vi "_exclude Event Structure Ref.vi"(1 "Part References":T2) -> (0 "NaN/Path/Refnum?":T1)   [LabVIEW 2014]
uses:
  <resource>/dialog/QuickDrop/plugins/_JKI State Machine Helper.llb/Part References -- Cluster__JKI_State_Machine_Helper.ctl
  <resource>/dialog/QuickDrop/plugins/_JKI State Machine Helper.llb/JKI SM__JKI_State_Machine_Helper.lvclass
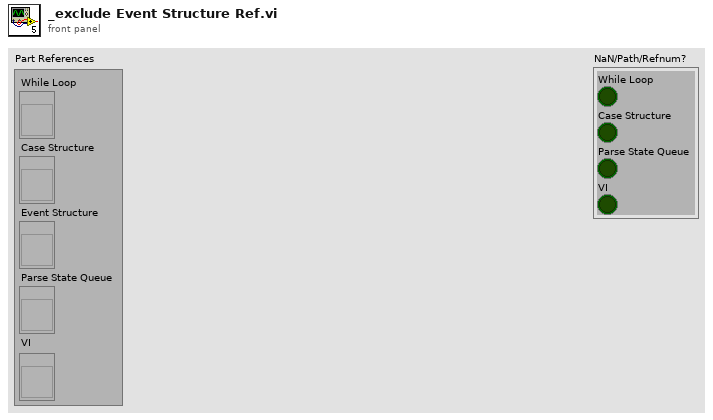
[diagram p1: front panel]
types:
  T1 = cluster{"While Loop":bool, "Case Structure":bool, "Parse State Queue":bool, "VI":bool}
  T2 = typedef "JKI State Machine API__JKI_State_Machine_Helper.lvlib/JKI SM__JKI_State_Machine_Helper.lvclass/Part References -- Cluster__JKI_State_Machine_Helper.ctl" = cluster{"While Loop":refnum<vi>, "Case Structure":refnum<vi>, "Event Structure":refnum<vi>, "Parse State Queue":refnum<vi>, "VI":refnum<vi>}
  T3 = cluster{"While Loop":refnum<vi>, "Case Structure":refnum<vi>, "Parse State Queue":refnum<vi>, "VI":refnum<vi>}
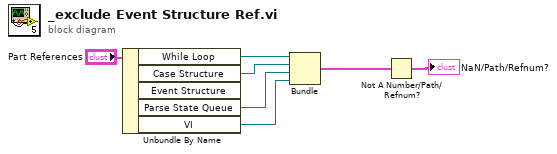
[diagram p0: block diagram]
diagram:
  n1 = Unbundle By Name("Part References") -> ("While Loop"=w6:refnum<vi>, "Case Structure"=w5:refnum<vi>, "Parse State Queue"=w4:refnum<vi>, "VI"=w3:refnum<vi>)  [unwired: 1 out]
  n2 = Bundle("While Loop"=w6, "Case Structure"=w5, "Parse State Queue"=w4, "VI"=w3) -> (w2:T3)  [unwired: 1 in]
  n3 = Not A Number/Path/Refnum?(number/path/refnum=w2) -> (NaN/Path/Refnum?=→"NaN/Path/Refnum?":T1)
